vi "Close Hardware.vi"(8 "error in (no error)":errorcluster, 11 "Inst.Xeryon-Rotator in":refnum<class "Inst.Xeryon-Rotator.lvclass">) -> (0 "error out":errorcluster, 3 "Inst.Xeryon-Rotator out":refnum<class "Inst.Xeryon-Rotator.lvclass">)   [LabVIEW 2019, in "Inst.Xeryon-Rotator.lvclass"]
uses:
  Inst.Xeryon-Rotator.lvclass
  Inst.Xeryon-Rotator.lvclass/Inst.Xeryon-Rotator.ctl
  <userlib>/LevyLab/Instrument Framework/Instrument Types/Cryostat/Instrument.Cryostat.lvclass
  drivers/Class/Controller/Controller.lvclass
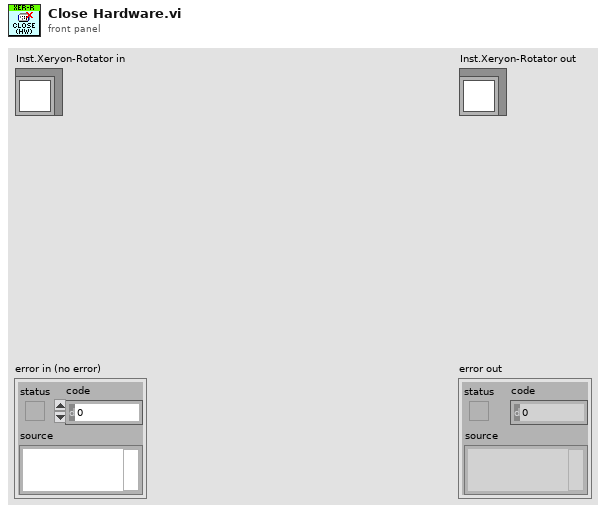
[diagram p1: front panel]
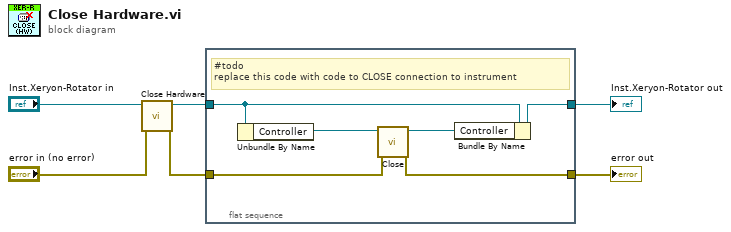
[diagram p0: block diagram]
diagram:
  n1 = call-parent "Close Hardware.vi"("error in (no error)"="error in (no error)", "Instrument in"="Inst.Xeryon-Rotator in") -> ("error out"=w4:errorcluster, "Instrument out"=w2:refnum<class "Inst.Xeryon-Rotator.lvclass">)  [unwired: 8 in]
  n2 = flat-sequence {
    tunnel: w4 -> [w7]
    tunnel: [w8] -> w3
    tunnel: w2 -> [w12]
    tunnel: [w11] -> w1
    frame #0 {
      # "#todo\nreplace this code with code to CLOSE connection to instrument"
      n3 = Unbundle By Name(w12) -> ("Controller"=w10:refnum<class "Controller.lvclass">)
      n4 = call-dynamic "Close.vi"("error in (no error)"=w7, "Controller in"=w10) -> ("error out"=w8:errorcluster, "Controller out"=w9:refnum<class "Controller.lvclass">)  [unwired: 8 in]
      n5 = Bundle By Name(cluster=w12, "Controller"=w9) -> (w11:refnum<class "Inst.Xeryon-Rotator.lvclass">)
    }
  }
  "error out" <- w3
  "Inst.Xeryon-Rotator out" <- w1
